vi "Refresh Layouts From VIs.vi"(8 "error in":errorcluster, 11 "state in":T1) -> (0 "error out":errorcluster, 3 "state out":T1)   [LabVIEW 2010, in "NI_SE_Config Front Panel Layout.lvlib"]
uses:
  NI_SE_Config Front Panel Layout.lvlib
  State.ctl
  VI Info.ctl
  VI Panel Layout/VI Panel Layout.lvclass
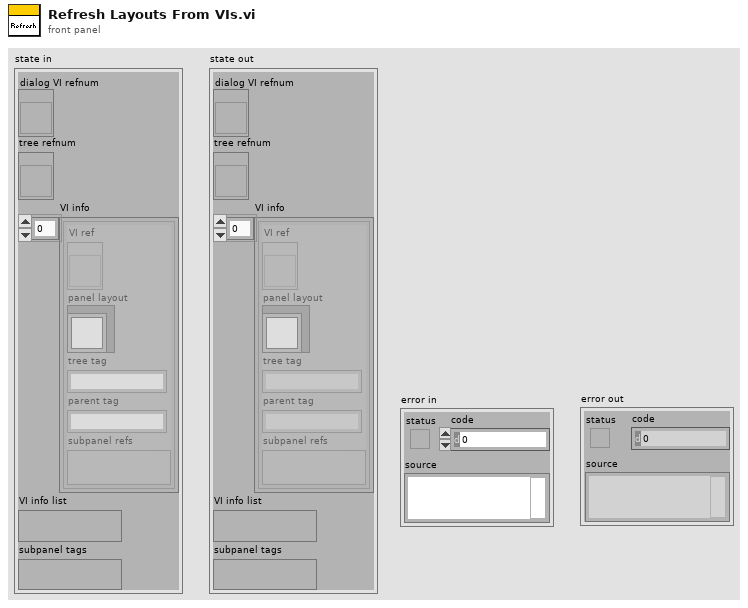
[diagram p1: front panel]
types:
  T1 = typedef "NI_SE_Config Front Panel Layout.lvlib/State.ctl" = cluster{"dialog VI refnum":refnum<vi>, "tree refnum":refnum<vi>, "VI info":T2[], "VI info list":variant, "subpanel tags":variant}
  T2 = typedef "NI_SE_Config Front Panel Layout.lvlib/VI Info.ctl" = cluster{"VI ref":refnum<vi>, "panel layout":refnum<class "VI Panel Layout.lvclass">, "tree tag":string, "parent tag":string, "subpanel refs":variant}
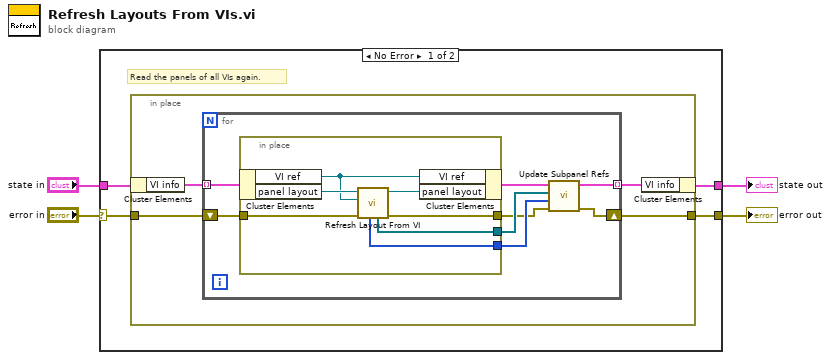
[diagram p0: block diagram]
diagram:
  n1 = case shown="No Error" "error in" {
    selector: "error in" -> [w7 w28]
    tunnel: "state in" -> [w8 w29]
    tunnel: [w5 w29] -> w2
    tunnel: [w6 w28] -> w1
    frame No Error {
      # "Read the panels of all VIs again."
      n2 = in-place {
        in-place-border: w7 -> [w10]
        in-place-border: [w9] -> w6
        n3 = in-place-cluster #1(w8) -> ("VI info"=w12:T2[])
        n4 = for {
          tunnel: w12 -> [w20] mode=indexing
          tunnel: [w17] -> w11 mode=indexing
          shift-right: [w14] -> w9
          shift-left: w10 -> [w19]
          n5 = in-place {
            in-place-border: [w24] -> w13
            in-place-border: w19 -> [w23]
            in-place-border: [w22] -> w16
            in-place-border: [w21] -> w15
            n6 = in-place-cluster #2(w20) -> ("VI ref"=w25:refnum<vi>, "panel layout"=w27:refnum<class "VI Panel Layout.lvclass">)
            n7 = call "Refresh Layout From VI.vi"("error in (no error)"=w23, "VI refnum"=w25, "VI Panel Layout in"=w27) -> ("error out"=w24:errorcluster, "VI Panel Layout out"=w26:refnum<class "VI Panel Layout.lvclass">, "subpanel refnums"=w22:refnum<vi>[], "subpanel UIDs"=w21:i32[])  [unwired: 5 in]
            n8 = in-place-cluster #2("VI ref"=w25, "panel layout"=w26) -> (w18:T2)
          }
          n9 = call "Update Subpanel Refs.vi"("error in"=w13, "subpanel UIDs"=w15, "subpanel refnums"=w16, "VI info in"=w18) -> ("error out"=w14:errorcluster, "VI info out"=w17:T2)  [unwired: 6 in]
        }
        n10 = in-place-cluster #1("VI info"=w11) -> (w5:T1)
      }
    }
    frame Error {
    }
  }
  "state out" <- w2
  "error out" <- w1
